vi "TSM DAQmx Relay Control.vi"(0 "TSM DAQmx Relay In":T1, 2 "Settling Time (s)":dbl, 5 "Relay Action":T3, 11 "error in":errorcluster) -> (15 "error out":errorcluster)   [LabVIEW 2019]
doc: "Performs the specified relay action on all specified relays."
uses:
  Pin Map/TSM DAQmx Relay Actions.ctl
  Pin Map/TSM DAQmx Relay.ctl
  <vilib>/NI_TestStand_SemiconductorModule/NI_TestStand_Semiconductor_Module.lvlibp/PinMap/General/SemiconductorModuleContext.ctl
  <vilib>/NI_TestStand_SemiconductorModule/NI_TestStand_Semiconductor_Module.lvlibp
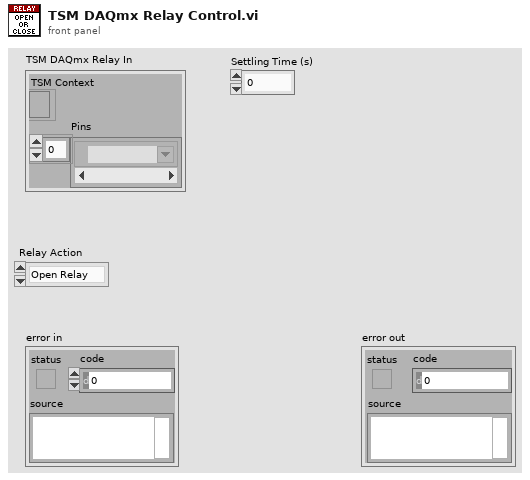
[diagram p1: front panel]
types:
  T1 = typedef "TSM DAQmx Relay.ctl" = cluster{"TSM Context":T2, "Pins":tag[]}
  T2 = typedef "NI_TestStand_Semiconductor_Module.lvlibp/SemiconductorModuleContext.ctl" = refnum<k7>
  T3 = typedef "TSM DAQmx Relay Actions.ctl" = enum16{"Open Relay", "Close Relay"}
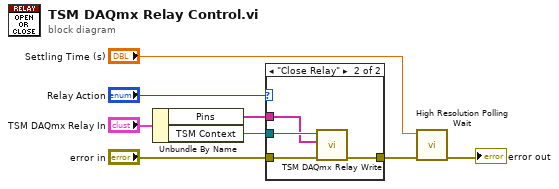
[diagram p0: block diagram]
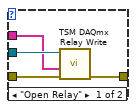
[diagram p2: hidden frame]
diagram:
  n1 = Unbundle By Name("TSM DAQmx Relay In") -> ("Pins"=w1:tag[], "TSM Context"=w3:T2)
  n2 = case shown="\"Close Relay\"" "Relay Action" {
    tunnel: "error in" -> [w12 w16]
    tunnel: [w11 w15] -> w4
    tunnel: w3 -> [w10 w14]
    tunnel: w1 -> [w9 w13]
    frame "Open Relay" {
      n3 = call "TSM DAQmx Relay Write.vi"("error in"=w12, "Pins to Output LOW"=w9, "TSM context in"=w10) -> ("error out"=w11:errorcluster)  [unwired: 7 in, 1 out]
    }
    frame "Close Relay" {
      n4 = call "TSM DAQmx Relay Write.vi"("error in"=w16, "Pins to Output HIGH"=w13, "TSM context in"=w14) -> ("error out"=w15:errorcluster)  [unwired: 7 in, 1 out]
    }
  }
  n5 = call <vilib>:"High Resolution Polling Wait.vi"("error in (no error)"=w4, "seconds to wait"="Settling Time (s)") -> ("error out"=→"error out":errorcluster)  [unwired: 9 in]
